vi "啮合 分离正反转.vi"(9 "输入扭矩":dbl[](array[numeric]), 11 "输入角度":dbl[](array[numeric])) -> (0 "扭矩反转":dbl[](array[numeric]), 1 "扭矩正转":dbl[](array[numeric]), 2 "角度反转":dbl[](array[numeric]), 3 "角度正转":dbl[](array[numeric]))   [LabVIEW 2015, in "Logging.lvlib"]
uses:
  Logging.lvlib
  <vilib>/Analysis/1siggen.llb/Ramp Pattern by Samples.vi
  <vilib>/gmath/NI_Gmath.lvlib
  <vilib>/Analysis/NI_AALBase.lvlib
panel:
  in  "细分因子":dbl=1.0
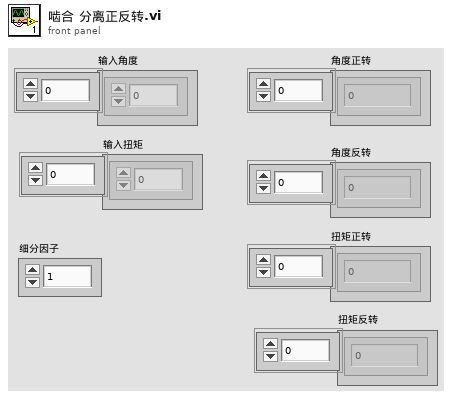
[diagram p1: front panel]
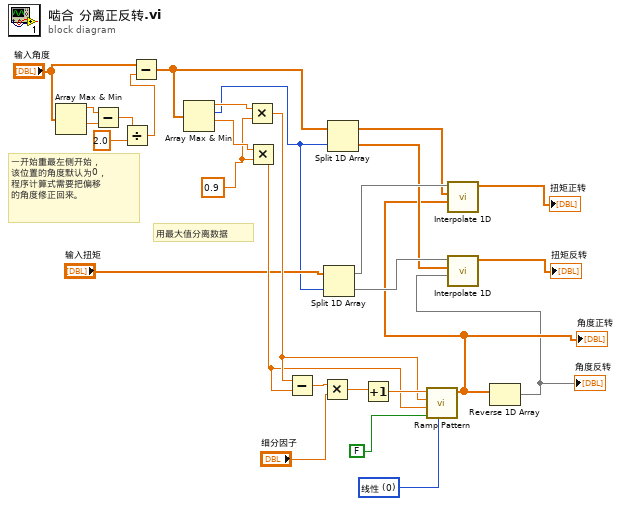
[diagram p0: block diagram]
diagram:
  w18 = u16 0 items=["线性", "对数"] ("type")
  w26 = 0.9 ("y")
  # "一开始重最左侧开始，\n该位置的角度默认为0，\n程序计算式需要把偏移\n的角度修正回来。"
  # "用最大值分离数据"
  n1 = Array Max & Min(array="输入角度") -> (max value=w6:dbl, min value=w7:dbl)  [unwired: 2 out]
  n2 = Subtract(x=w6, y=w7) -> (x-y=w5:dbl)
  n3 = Divide(x=w5, y=2.0) -> (x/y=w2:dbl)
  n4 = Subtract(x="输入角度", y=w2) -> (x-y=w1:dbl[])
  n5 = Array Max & Min(array=w1) -> (max value=w28:dbl, max index (indices)=w16:i32, min value=w27:dbl)  [unwired: 1 out]
  n6 = Multiply(x=w28, y=w26) -> (x*y=w21:dbl)
  n7 = Multiply(x=w27, y=w26) -> (x*y=w20:dbl)
  n8 = Subtract(x=w21, y=w20) -> (x-y=w22:dbl)
  n9 = Multiply(x=w22, y="细分因子") -> (x*y=w25:dbl)
  n10 = Split 1D Array(array="输入扭矩", index=w16) -> (first subarray=w15:dbl[], second subarray=w13:dbl[])
  n11 = Split 1D Array(array=w1, index=w16) -> (first subarray=w14:dbl[], second subarray=w12:dbl[])
  n12 = Increment(x=w25) -> (x+1=w24:dbl)
  n13 = call-poly <vilib>:"Ramp Pattern.vi"("type"=w18, "exclude end?"=FALSE, "start"=w20, "end"=w21, "samples"=w24) -> ("Ramp Pattern"=w9:dbl[])  [unwired: 5 in, 1 out]
  "角度正转" <- w9
  n14 = call <vilib>:"Interpolate 1D.vi"("xi"=w9, "X"=w14, "Y"=w15) -> ("yi"=→"扭矩正转":dbl[])  [unwired: 6 in, 2 out]
  n15 = Reverse 1D Array(array=w9) -> (reversed array=w8:dbl[])
  "角度反转" <- w8
  n16 = call <vilib>:"Interpolate 1D.vi"("xi"=w8, "X"=w12, "Y"=w13) -> ("yi"=→"扭矩反转":dbl[])  [unwired: 6 in, 2 out]
